vi "DUTResultsDialog.vi"(5 "Left Coordinate":i16, 7 "Top Coordinate":i16, 8 "error in (no error)":errorcluster, 9 "MessageTxt":string, 10 "TestSocketIndex":i32, 11 "Value":string) -> (0 "error out":errorcluster)   [LabVIEW 2019]
doc: "Display DUT results banner for Pass, Fail, Error or Terminate."
panel:
  out "MssgText":string
  out "Message":string
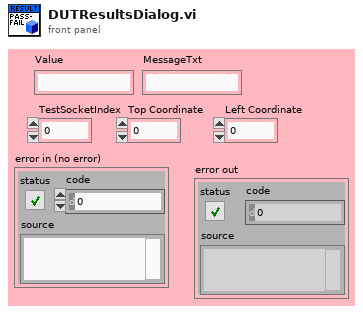
[diagram p1: front panel]
types:
  T1 = typedef "imagedata.ctl" = cluster{"image type":i32, "image depth":i32, "image":u8[], "mask":u8[], "colors":u32[], "Rectangle":cluster{"left":i16, "top":i16, "right":i16, "bottom":i16}}
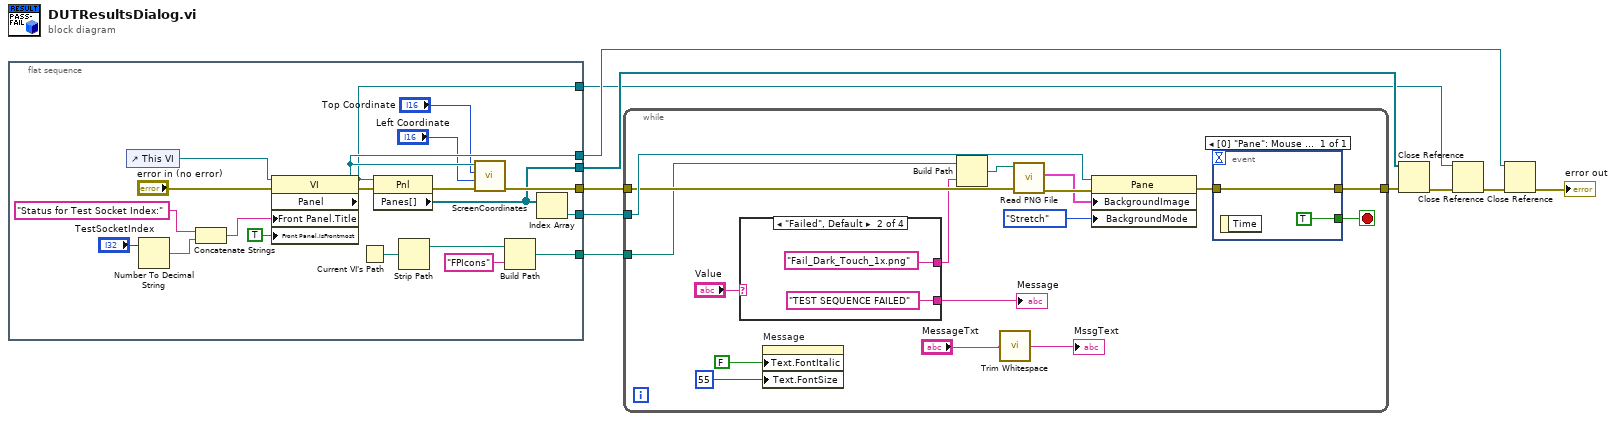
[diagram p0: block diagram]
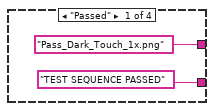
[diagram p2: hidden frame]
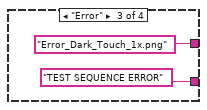
[diagram p3: hidden frame]
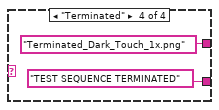
[diagram p4: hidden frame]
diagram:
  n1 = flat-sequence {
    tunnel: [w30] -> w8
    tunnel: [w24] -> w2
    tunnel: [w18] -> w7
    tunnel: [w15] -> w6
    tunnel: [w13] -> w5
    tunnel: [w12] -> w1
    frame #0 {
      n2 = control-ref of="This VI"() -> (w21:refnum<vi>)
      n3 = Number To Decimal String(number="TestSocketIndex") -> (decimal integer string=w25:string)  [unwired: 1 in]
      n4 = Concatenate Strings("Status for Test Socket Index:", w25) -> (w20:string)
      n5 = property class="VI"(reference=w21, error in="error in (no error)", "Front Panel.Title"=w20, "Front Panel.IsFrontmost"=TRUE ("Front Panel Window:Is Frontmost")) -> (reference out=w24:refnum<vi>, error out=w27:errorcluster, "Panel"=w12:refnum<vi>)
      n6 = Current VI's Path() -> (path=w17:path)
      n7 = property class="Pnl"(reference=w12, error in=w27) -> (error out=w19:errorcluster, "Panes[]"=w13:refnum<vi>[])  [unwired: 1 out]
      n8 = Strip Path(path=w17) -> (stripped path=w14:path)  [unwired: 1 out]
      n9 = call "ScreenCoordinates.vi"("error in (no error)"=w19, "Left Coordinate"="Left Coordinate", "Top Coordinate"="Top Coordinate", "ThisVI"=w24) -> ("error out"=w30:errorcluster)  [unwired: 6 in, 1 out]
      n10 = Build Path(base path=w14, name or relative path="FPIcons") -> (appended path=w15:path)
      n11 = Index Array(array=w13) -> (element=w18:refnum<vi>)  [unwired: 1 in]
    }
  }
  n12 = while {
    tunnel: [w34] -> w10
    tunnel: w8 -> [w42]
    tunnel: w7 -> [w44]
    tunnel: w6 -> [w38]
    stop <- w33 stop-if-true
    n13 = case shown="\"Failed\", Default" "Value" {
      tunnel: ["TEST SEQUENCE PASSED" "TEST SEQUENCE FAILED" "TEST SEQUENCE ERROR" "TEST SEQUENCE TERMINATED"] -> w40
      tunnel: ["Pass_Dark_Touch_1x.png" "Fail_Dark_Touch_1x.png" "Error_Dark_Touch_1x.png" "Terminated_Dark_Touch_1x.png"] -> w37
      frame "Passed" {
      }
      frame "Failed", Default {
      }
      frame "Error" {
      }
      frame "Terminated" {
      }
    }
    "Message" <- w40
    n14 = property on="Message" class="Str"("Text.FontItalic"=FALSE ("Text.Font:Bold"), "Text.FontSize"=u32 55 ("Text.Font:Size")) -> ()  [unwired: 2 in, 2 out]
    n15 = Build Path(base path=w38, name or relative path=w37) -> (appended path=w36:path)
    n16 = call <vilib>:"Trim Whitespace.vi"("string"="MessageTxt") -> ("trimmed string"=→"MssgText":string)  [unwired: 1 in]
    n17 = call <vilib>:"Read PNG File.vi"("error in (no error)"=w42, "path to PNG file"=w36) -> ("error out"=w41:errorcluster, "image data"=w39:T1)  [unwired: 7 in, 1 out]
    n18 = property class="Pane"(reference=w44, error in=w41, "BackgroundImage"=w39, "BackgroundMode"=enum16{"Stretch", "Center", "Tile"}."Stretch" ("Background Mode")) -> (error out=w35:errorcluster)  [unwired: 1 out]
    n19 = event shown="[0] \"Pane\": Mouse Down" {
      selector: _ -> [_]
      dyn-events: _ -> [_]
      timeout: _ -> [_]
      tunnel: w35 -> [w49]
      tunnel: [w49] -> w34
      tunnel: [TRUE] -> w33
      event Mouse Down {
        n20 = event-data() -> ()  [unwired: 1 in, 1 out]
      }
    }
  }
  n21 = Close Reference(reference=w5, error in (no error)=w10) -> (error out=w9:errorcluster)
  n22 = Close Reference(reference=w1, error in (no error)=w9) -> (error out=w4:errorcluster)
  n23 = Close Reference(reference=w2, error in (no error)=w4) -> (error out=→"error out":errorcluster)
